vi "Plot Waveform Cluster.vi"(6 "Line Plot Config":T1, 7 "Save path":path=path "C:/Users/bogum/OneDrive/Dokumenty/Git/LabVIEW Python Ploter/LabVIEW_python_ploter.py", 8 "error in (no error)":errorcluster, 10 "Waveform":waveform(dbl), 11 "PythonPlotter in":refnum<class "PythonPlotter.lvclass">) -> (0 "error out":errorcluster, 3 "PythonPlotter out":refnum<class "PythonPlotter.lvclass">)   [LabVIEW 2024, in "PythonPlotter.lvclass"]
uses:
  PythonPlotter.lvclass
  PythonPlotter.lvclass/PythonPlotter.ctl
  <vilib>/Analysis/NI_AALBase.lvlib
  <vilib>/Analysis/1siggen.llb/Ramp Pattern by Samples.vi
  #linePlotConfig.ctl
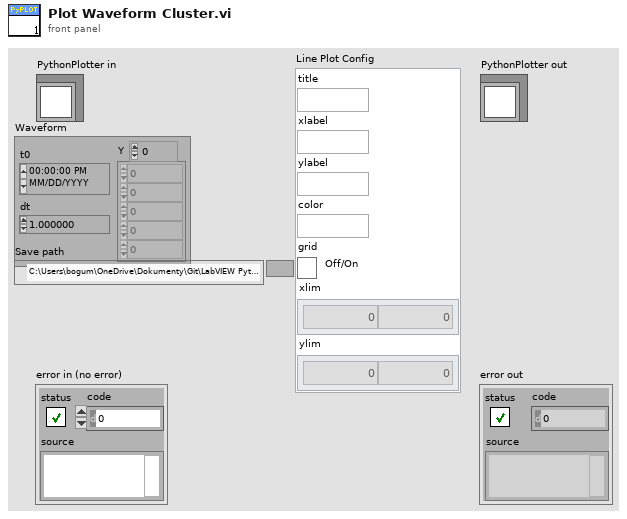
[diagram p1: front panel]
types:
  T1 = typedef "PythonPlotter.lvclass/#linePlotConfig.ctl" = cluster{"title":string, "xlabel":string, "ylabel":string, "color":string, "grid":bool, "xlim":dbl[], "ylim":dbl[]}
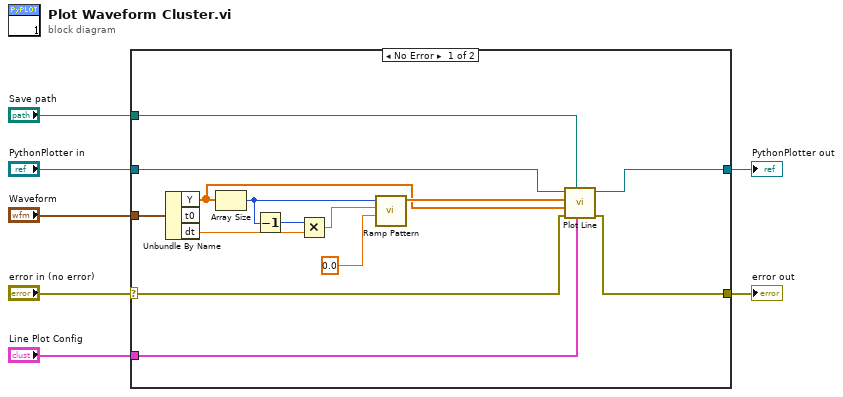
[diagram p0: block diagram]
diagram:
  n1 = case shown="No Error" "error in (no error)" {
    selector: "error in (no error)" -> [w11 w23]
    tunnel: [w10 w23] -> w6
    tunnel: [w13 w22] -> w4
    tunnel: "PythonPlotter in" -> [w14 w22]
    tunnel: "Waveform" -> [w21 _]
    tunnel: "Save path" -> [w12 _]
    tunnel: "Line Plot Config" -> [w8 _]
    frame No Error {
      n2 = Unbundle By Name(w21) -> ("Y"=w9:dbl[], "dt"=w18:dbl)  [unwired: 1 out]
      n3 = Array Size(array=w9) -> (size(s)=w19:i32)
      n4 = Decrement(x=w19) -> (x-1=w15:i32)
      n5 = Multiply(x=w15, y=w18) -> (x*y=w17:dbl)
      n6 = call-poly <vilib>:"Ramp Pattern.vi"("start"=0.0, "end"=w17, "samples"=w19) -> ("Ramp Pattern"=w16:dbl[])  [unwired: 7 in, 1 out]
      n7 = call "Plot Line.vi"("Line Plot Config"=w8, "Save path"=w12, "error in (no error)"=w11, "Y"=w9, "X"=w16, "PythonPlotter in"=w14) -> ("error out"=w10:errorcluster, "PythonPlotter out"=w13:refnum<class "PythonPlotter.lvclass">)  [unwired: 4 in]
    }
    frame Error {
    }
  }
  "error out" <- w6
  "PythonPlotter out" <- w4
